vi "mcl -- read v1.vi"() -> ()   [LabVIEW 2019]
uses:
  nanocal/Nanocalorimetry/data/MCL.lvlibp/SynkTek Host/LIdata/LIData_SelectReadingType.ctl
  nanocal/Nanocalorimetry/data/MCL.lvlibp/SynkTek FPGA/FPGA_SharedResources/FPGASharedResources_Readings_ReadingChannelTypedef.ctl
  nanocal/Nanocalorimetry/data/MCL.lvlibp/SynkTek FPGA/FPGA_SharedResources/FPGASharedResources_PhaseType_Typedef.ctl
  nanocal/Nanocalorimetry/data/MCL.lvlibp/SynkTek FPGA/FPGA_SharedResources/FPGASharedResources_Lockin_Typedef.ctl
  nanocal/Nanocalorimetry/data/MCL.lvlibp
  nanocal/Nanocalorimetry/data/MCL.lvlibp/SynkTek FPGA/FPGA_SharedResources/FPGA_SharedResources.lvlib
  nanocal/Nanocalorimetry/data/MCL.lvlibp/SynkTek Host/LIdata/LIData.lvlib
panel:
  out "Select Readings":dbl[](array[numeric])
  in  "Reading types":T1[](array[typedef])
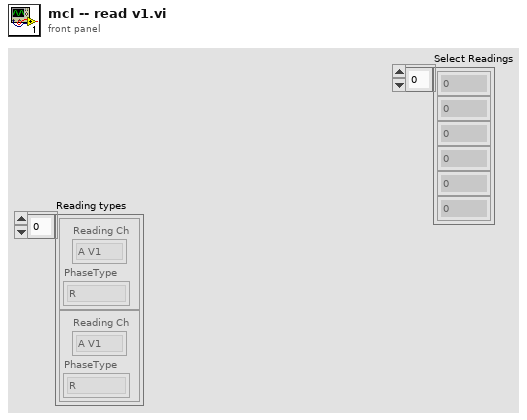
[diagram p1: front panel]
types:
  T1 = typedef "MCL.lvlibp/LIData.lvlib/LIData_SelectReadingType.ctl" = cluster{"Reading Ch":T2, "PhaseType":T3}
  T2 = typedef "MCL.lvlibp/FPGA_SharedResources.lvlib/FPGASharedResources_Readings_ReadingChannelTypedef.ctl" = enum8{"A V1", "A V2", "B V1", "B V2", "C V1", "C V2", "D V1", "D V2", "E V1", "E V2", "A I", "B I", "C I", "D I", "E I", "Int."}
  T3 = typedef "MCL.lvlibp/FPGA_SharedResources.lvlib/FPGASharedResources_PhaseType_Typedef.ctl" = enum16{"DC", "X", "Y", "R", "Theta"}
  T4 = typedef "MCL.lvlibp/FPGA_SharedResources.lvlib/FPGASharedResources_Lockin_Typedef.ctl" = enum8{"Lock-in set L1", "Lock-in set L2"}
  T5 = typedef "MCL.lvlibp/MCL_DataRef.ctl" = refnum<vi>
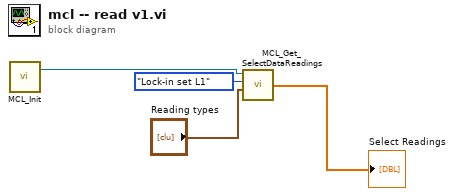
[diagram p0: block diagram]
diagram:
  n1 = call "MCL_Init.vi"() -> ("MCL object"=w4:T5)  [unwired: 2 in, 1 out]
  n2 = call "MCL_Get_SelectDataReadings.vi"("Reading types"="Reading types", "Lockin"=FPGASharedResources_Lockin_Typedef."Lock-in set L1", "MCL object"=w4) -> ("Select Readings"=→"Select Readings":dbl[])  [unwired: 1 in, 2 out]
